vi "DisclaimerTest.vi"() -> ()   [LabVIEW 2020]
panel:
  in  "Stop":bool
  out "Numeric":i32
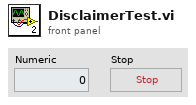
[diagram p1: front panel]
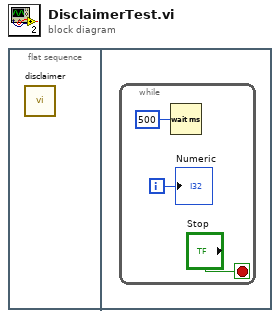
[diagram p0: block diagram]
diagram:
  n1 = flat-sequence {
    frame #0 {
      n2 = call "disclaimer.vi"() -> ()  [unwired: 12 in]
    }
    frame #1 {
      n3 = while {
        i -> [w2]
        stop <- "Stop" stop-if-true
        n4 = Wait (ms)(milliseconds to wait=u32 500) -> ()  [unwired: 1 out]
        "Numeric" <- w2
      }
    }
  }
